vi "calibration function H2O.vi"(7 "x":dbl) -> (8 "f(x)":dbl)   [LabVIEW 2010, in "LicorLI7000.lvlib"]
uses:
  LicorLI7000.lvlib
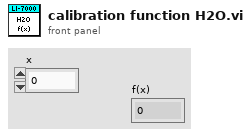
[diagram p1: front panel]
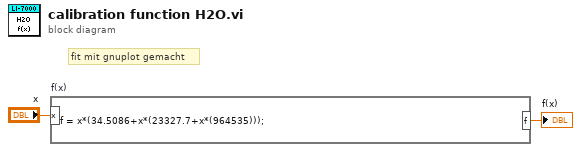
[diagram p0: block diagram]
diagram:
  # "fit mit gnuplot gemacht"
  n1 = formula code="f = x*(34.5086+x*(23327.7+x*(964535)));" "f(x)"("x"="x") -> ("f"=→"f(x)":dbl)
